vi "Discover Spectrum Analyzer Model.vi"(10 "Model In":string) -> (2 "selection":bool)   [LabVIEW 2018]
panel:
  out "size(s)":i32
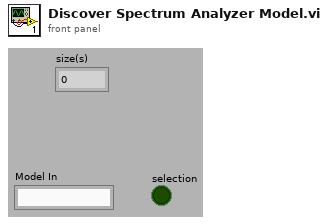
[diagram p1: front panel]
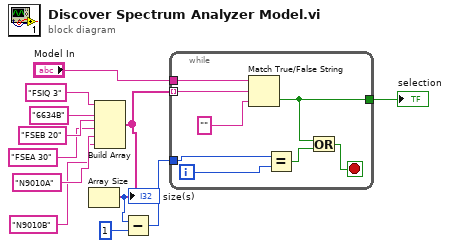
[diagram p0: block diagram]
diagram:
  n1 = Build Array("FSIQ 3" ("true string"), "6634B" ("true string"), "FSEB 20" ("element"), "FSEA 30" ("element"), "N9010A" ("element"), "N9010B" ("element")) -> (w8:string[])
  n2 = Array Size(array=w8) -> (size(s)=w7:i32)
  "size(s)" <- w7
  n3 = Subtract(x=w7, y=1) -> (x-y=w5:i32)
  n4 = while {
    tunnel: w8 -> [w19] mode=indexing
    tunnel: "Model In" -> [w18]
    tunnel: [w17] -> w9
    tunnel: w5 -> [w13]
    i -> [w14]
    stop <- w16 stop-if-true
    n5 = Match True/False String(2:"" ("false string"), 3:w19, 4:w18) -> (0:w17:bool)  [unwired: 1 out]
    n6 = Equal?(x=w13, y=w14) -> (x = y?=w15:bool)
    n7 = Or(x=w17, y=w15) -> (x .or. y?=w16:bool)
  }
  "selection" <- w9
